vi "9219_UpdateConfigBox.vi"(10 "9219 Data in":T1 {"Conversion Time" items=["High Speed", "Best 60 Hz Rejection", "Best 50 Hz Rejection", "High Resolution"]; "TCoupleType" items=["J", "K", "T", "E", "R", "S", "N", "B"]; "DegreeRange" items=["Raw units", "Degrees Kelvin", "Degrees Celsius", "Degrees Fahrenheit", "Degrees Rankine"]; "RtdType" items=["TCR3851"=1, "TCR3750"=2, "TCR3916"=3, "TCR3920"=4, "TCR3911"=5, "TCR3928"=6, "Custom"=0]}, 11 "Channel Refnum":refnum<vi>) -> ()   [LabVIEW 2011, in "Modules.lvlib" / "9219.lvclass"]
uses:
  9219.lvclass
  9219 Config.ctl
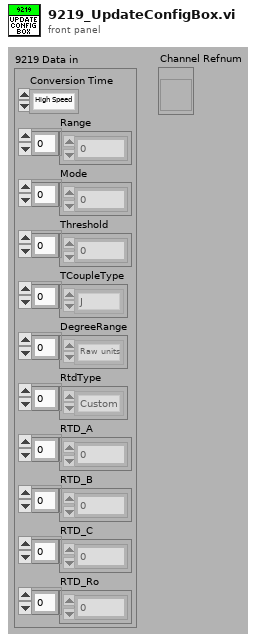
[diagram p1: front panel]
types:
  T1 = typedef "Modules.lvlib/9219.lvclass/9219 Config.ctl" = cluster{"Conversion Time":u16, "Range":u8[], "Mode":u8[], "Threshold":dbl[], "TCoupleType":u8[], "DegreeRange":u8[], "RtdType":u8[], "RTD_A":dbl[], "RTD_B":dbl[], "RTD_C":dbl[], "RTD_Ro":dbl[]}
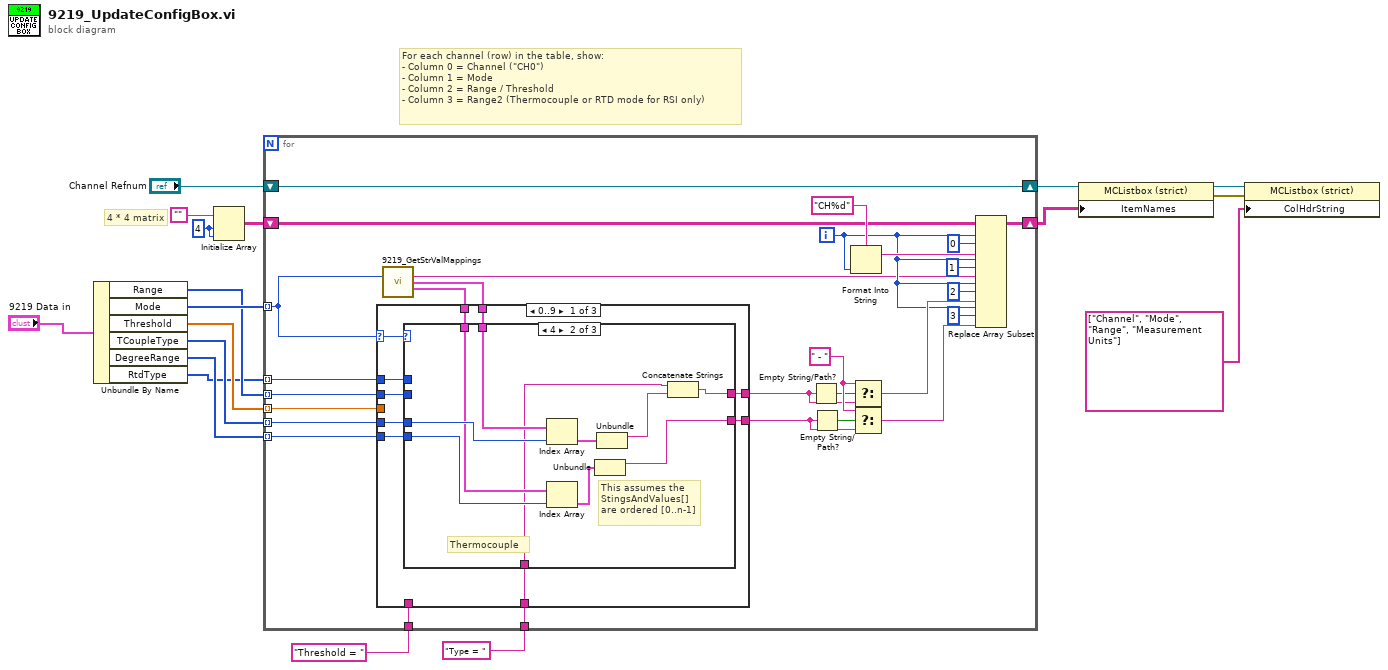
[diagram p0: block diagram]
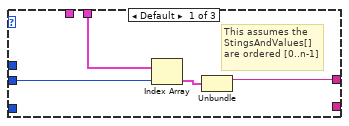
[diagram p2: hidden frame]
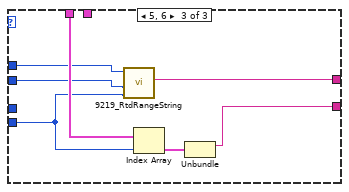
[diagram p3: hidden frame]
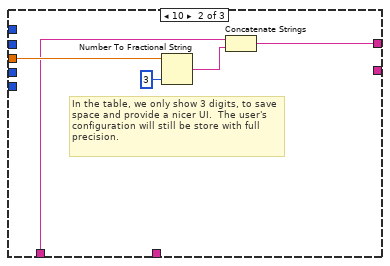
[diagram p4: hidden frame]
diagram:
  w17 = 4 ("dimension size")
  # "For each channel (row) in the table, show:\n- Column 0 = Channel (\"CH0\")\n- Column 1 = Mode\n- Column 2 = Range / Threshold\n- Column 3 = Range2 (Thermocouple or RTD mode for RSI only)"
  # "4 * 4 matrix"
  n1 = Unbundle By Name("9219 Data in") -> ("Range"=w9:u8[], "Mode"=w13:u8[], "Threshold"=w10:dbl[], "TCoupleType"=w11:u8[], "DegreeRange"=w12:u8[], "RtdType"=w8:u8[])
  n2 = Initialize Array("", w17, w17) -> (w15:string[][])
  n3 = for {
    shift-right: [w40] -> w4
    shift-left: w15 -> [w33]
    shift-right: [w19] -> w5
    shift-left: "Channel Refnum" -> [w19]
    tunnel: w13 -> [w23] mode=indexing
    tunnel: w12 -> [w32] mode=indexing
    tunnel: w11 -> [w31] mode=indexing
    tunnel: w10 -> [w30] mode=indexing
    tunnel: w9 -> [w29] mode=indexing
    tunnel: w8 -> [w28] mode=indexing
    tunnel: "Threshold = " ("String") -> [w27]
    tunnel: "Type = " ("String") -> [w26]
    i -> [w34]
    w39 = " - "
    n4 = call "9219_GetStrValMappings.vi"("_Mode"=w23) -> ("_Mode (str)"=w20:string, "_Range Strings And Values []"=w21:cluster{"String":string, "Value":u16}[], "_Range2 Strings And Values []"=w22:cluster{"String":string, "Value":u16}[])  [unwired: 11 in, 1 out]
    n5 = case shown="0..9" w23 {
      selector: w23 -> [w54 _ _]
      tunnel: w29 -> [w55 _ _]
      tunnel: w30 -> [_ w82 _]
      tunnel: w21 -> [w56 _ _]
      tunnel: w32 -> [w53 _ _]
      tunnel: w31 -> [w52 _ _]
      tunnel: w22 -> [w51 _ _]
      tunnel: [w49 w80 _] -> w25
      tunnel: [w50 _ _] -> w24
      tunnel: w28 -> [w48 _ _]
      tunnel: w26 -> [w47 _ _]
      tunnel: w27 -> [_ w78 _]
      frame 0..9 {
        n6 = case shown="4" w54 {
          tunnel: w56 -> [w59 w70 _]
          tunnel: w55 -> [w58 _ w72]
          tunnel: w53 -> [_ w69 w71]
          tunnel: w52 -> [_ w68 _]
          tunnel: w51 -> [_ w67 w77]
          tunnel: [_ w66 w76] -> w50
          tunnel: [w57 w65 w74] -> w49
          tunnel: w48 -> [_ _ w73]
          tunnel: w47 -> [_ w64 _]
          frame Default {
            # "This assumes the StingsAndValues[] are ordered [0..n-1]"
            n7 = Index Array(array=w59, index=w58) -> (element=w60:cluster{"String":string, "Value":u16})
            n8 = Unbundle(w60) -> ("String"=w57:string)  [unwired: 1 out]
          }
          frame 4 {
            # "This assumes the StingsAndValues[] are ordered [0..n-1]"
            # "Thermocouple"
            n9 = Index Array(array=w70, index=w68) -> (element=w63:cluster{"String":string, "Value":u16})
            n10 = Index Array(array=w67, index=w69) -> (element=w62:cluster{"String":string, "Value":u16})
            n11 = Unbundle(w62) -> ("String"=w66:string)  [unwired: 1 out]
            n12 = Unbundle(w63) -> ("String"=w61:string)  [unwired: 1 out]
            n13 = Concatenate Strings(w64, w61) -> (w65:string)
          }
          frame 5, 6 {
            n14 = call "9219_RtdRangeString.vi"("_Degree Range"=w71, "_Range"=w72, "RTD Type"=w73) -> ("_RTD String"=w74:string)  [unwired: 8 in]
            n15 = Index Array(array=w77, index=w71) -> (element=w75:cluster{"String":string, "Value":u16})
            n16 = Unbundle(w75) -> ("String"=w76:string)  [unwired: 1 out]
          }
        }
      }
      frame 10 {
        # "In the table, we only show 3 digits, to save space and provide a nicer UI.  The user's configuration will still be store with full precision."
        n17 = Number To Fractional String(number=w82, precision (6)=i16 3) -> (F-format string=w81:string)  [unwired: 2 out]
        n18 = Concatenate Strings(w78, w81) -> (w80:string)
      }
      frame 11, Default {
      }
    }
    n19 = Empty String/Path?(string/path=w25) -> (empty?=w37:bool)
    n20 = Empty String/Path?(string/path=w24) -> (empty?=w38:bool)
    n21 = Format Into String(format string="CH%d", w34) -> (resulting string=w45:string)  [unwired: 2 in, 1 out]
    n22 = Select(t=w39, s=w37, f=w25) -> (s? t:f=w35:string)
    n23 = Select(t=w39, s=w38, f=w24) -> (s? t:f=w36:string)
    n24 = Replace Array Subset(array=w33, new element #1=w45, index (row) #1=w34, index (col) #1=0 ("Column 1"), new element #2=w20, index (row) #2=w34, index (col) #2=1 ("Column 1"), new element #3=w35, index (row) #3=w34, index (col) #3=2 ("disabled index (col)"), new element #4=w36, index (row) #4=w34, index (col) #4=3 ("disabled index (col)")) -> (w40:string[][])
  }
  n25 = property on="Property Node" class="MCListbox (strict)"(reference=w5, "ItemNames"=w4) -> (reference out=w3:refnum<vi>, error out=w2:errorcluster)  [unwired: 1 in]
  n26 = property on="Property Node" class="MCListbox (strict)"(reference=w3, error in=w2, "ColHdrString"=string[] ["Channel", "Mode", "Range", "Measurement Units"] ("Column Header Strings[]")) -> ()  [unwired: 2 out]
